vi "Open Font.vi"(8 "error in (no error)":errorcluster, 10 "Size":i32, 11 "File":path) -> (0 "error out":errorcluster, 3 "Font Pointer":u32 format="%.0x")   [LabVIEW 2015, in "LibSDL2_TTF.lvlib"]
uses:
  LibSDL2_TTF.lvlib
  LibSDL2 Wrapper/DLL/SDL2_ttf.dll
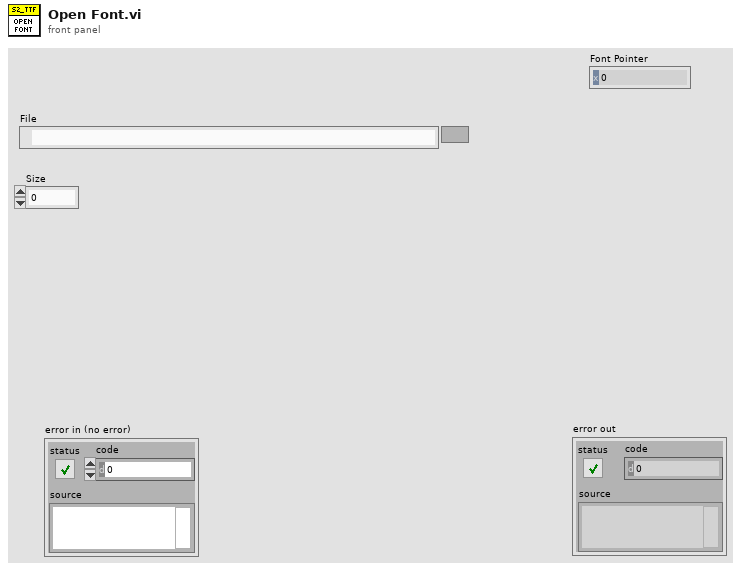
[diagram p1: front panel]
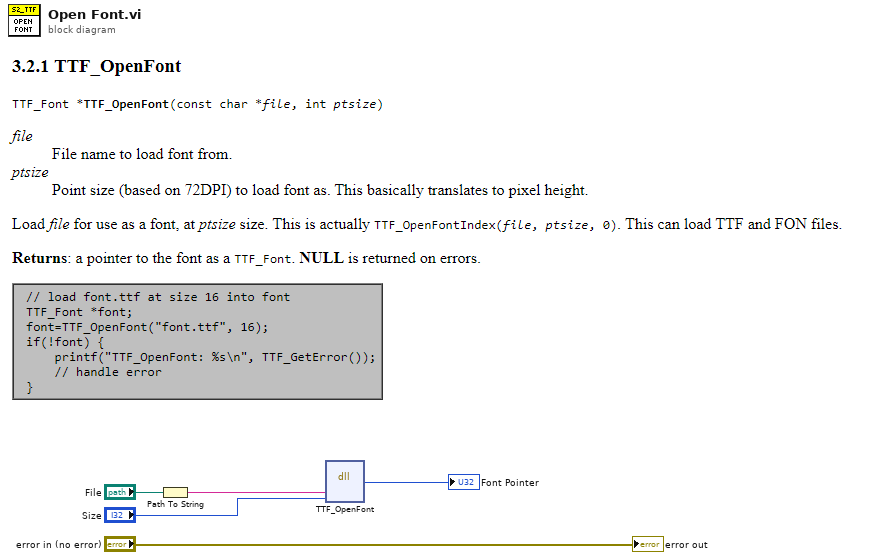
[diagram p0: block diagram]
diagram:
  n1 = Path To String(path="File") -> (string=w3:string)
  n2 = dll-call lib="C:/dev/PGS/LabSDL2/Source/Libraries/LibSDL2 Wrapper/DLL/SDL2_ttf.dll" fn="TTF_OpenFont"("File"=w3, "Size"="Size") -> ("Font Pointer"=→"Font Pointer":u32)  [unwired: 5 in, 2 out]
  "error out" <- "error in (no error)"
